vi "Connect.vi"(8 "error in (no error)":errorcluster, 11 "VideoScanCamera in":refnum<class "VideoScanDeviceLibrary.lvclass">) -> (0 "error out":errorcluster, 3 "VideoScanCamera out":refnum<class "VideoScanDeviceLibrary.lvclass">)   [LabVIEW 2014, in "VideoScanDeviceLibrary.lvclass"]
uses:
  VideoScanDeviceLibrary.lvclass
  VideoScanDeviceLibrary.lvclass/VideoScanDeviceLibrary.ctl
  <vilib>/MediaMongrels Ltd/WebSockets/WebSockets/WebSockets.lvlib
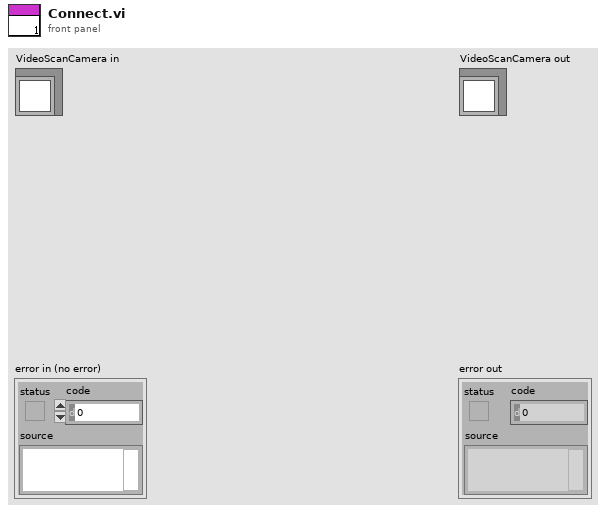
[diagram p1: front panel]
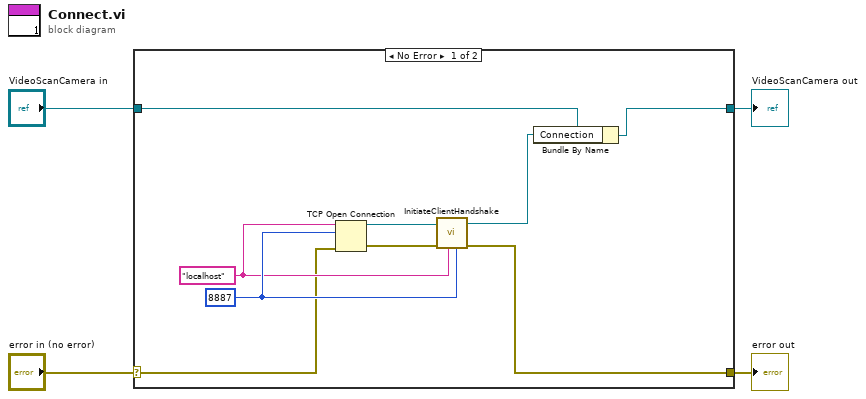
[diagram p0: block diagram]
diagram:
  n1 = case shown="No Error" "error in (no error)" {
    selector: "error in (no error)" -> [w6 w15]
    tunnel: [w5 w15] -> w3
    tunnel: [w8 w14] -> w1
    tunnel: "VideoScanCamera in" -> [w9 w14]
    frame No Error {
      w11 = "localhost" ("name")
      w12 = u16 8887 ("port")
      n2 = TCP Open Connection(address=w11, remote port or service name=w12, error in (no error)=w6) -> (connection ID=w13:refnum<k5>, error out=w10:errorcluster)  [unwired: 2 in]
      n3 = call <vilib>:"InitiateClientHandshake.vi"("remote port or service name"=w12, "address ('localhost')"=w11, "error in (no error)"=w10, "WebSocket Connection in"=w13) -> ("error out"=w5:errorcluster, "WebSocket Connection out"=w7:refnum<k5>)  [unwired: 5 in, 1 out]
      n4 = Bundle By Name(cluster=w9, "Connection"=w7) -> (w8:refnum<class "VideoScanDeviceLibrary.lvclass">)
    }
    frame Error {
    }
  }
  "error out" <- w3
  "VideoScanCamera out" <- w1
